vi "Remove Package Dialog.vi"(8 "error in (no error)":errorcluster, 11 "removed package filepath":path) -> (0 "error out":errorcluster)   [LabVIEW 2014]
doc: "Launches a dialog to confirm unpublishing a package from a feed and ask whether to delete the package file (.nipkg)"
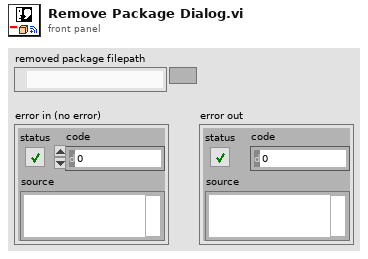
[diagram p1: front panel]
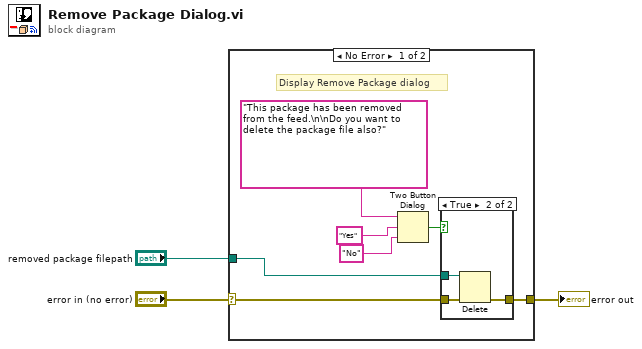
[diagram p0: block diagram]
diagram:
  n1 = case shown="No Error" "error in (no error)" {
    selector: "error in (no error)" -> [w10 w15]
    tunnel: [w6 w15] -> w1
    tunnel: "removed package filepath" -> [w4 _]
    frame No Error {
      # "Display Remove Package dialog"
      n2 = Two Button Dialog(message="This package has been removed from the feed.\n\nDo you want to delete the package file also?", 1:"No" ("F button name (\"Cancel\")"), 2:"Yes" ("T button name (\"OK\")")) -> (T button?=w5:bool)
      n3 = case shown="True" w5 {
        tunnel: w10 -> [w11 w14]
        tunnel: [w11 w13] -> w6
        tunnel: w4 -> [_ w12]
        frame False {
        }
        frame True {
          n4 = Delete(path (use dialog)=w12, error in=w14) -> (error out=w13:errorcluster)  [unwired: 3 in, 2 out]
        }
      }
    }
    frame Error {
    }
  }
  "error out" <- w1
